vi "jsonToLibera.vi"(0 "json":string, 2 "Enable ADC SP":bool, 5 "Enable DD":bool, 7 "Enable SA":bool, 9 "Enable ADC CW":bool, 13 "Enable AVG":bool) -> (1 "ADC_CW":T1(array[cluster]), 3 "DD":T5(array[cluster]), 4 "mode":i32, 6 "acquisitions":string, 8 "libera_error":i32, 10 "samples":i32, 11 "STATUS":string, 12 "AVG":cluster{"AVG":i32}[](array[cluster]), 14 "SA":T3(array[cluster]), 15 "ADC_SP":T2(array[cluster]))   [LabVIEW 2012]
uses:
  chaos-common-crest/LabVIEW/LV14/chaosui-crest/chaosui-crest.lvlib
panel:
  out "value":T4
  out "nok":i32
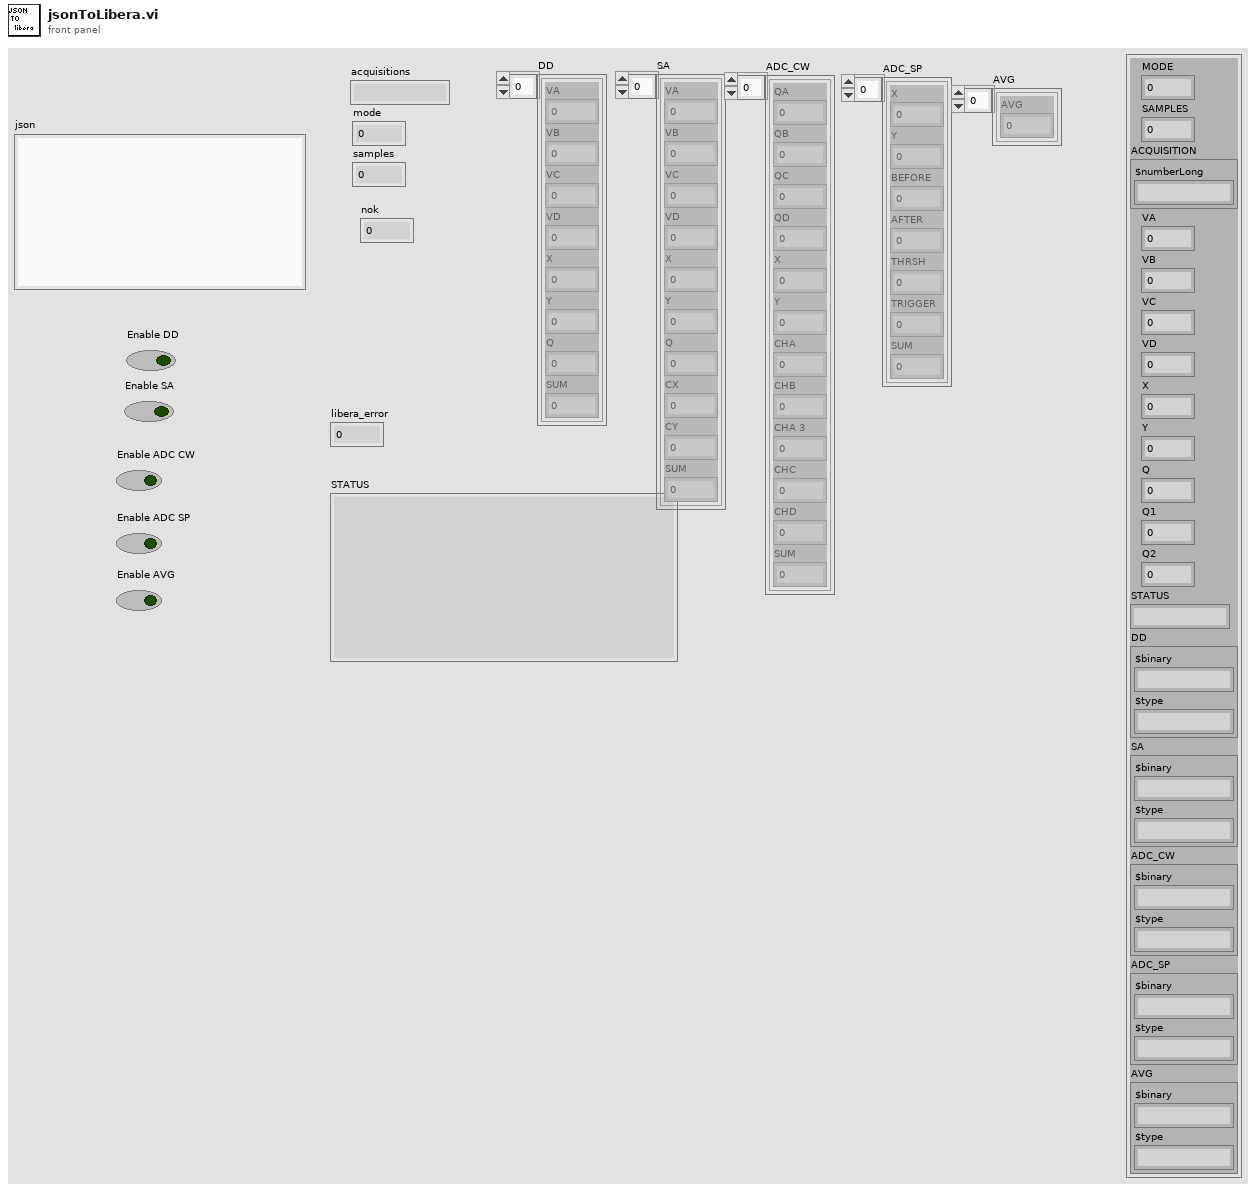
[diagram p1: front panel]
types:
  T1 = cluster{"QA":i32, "QB":i32, "QC":i32, "QD":i32, "X":i32, "Y":i32, "CHA":i32, "CHB":i32, "CHA 3":i32, "CHC":i32, "CHD":i32, "SUM":i32}[]
  T2 = cluster{"X":i32, "Y":i32, "BEFORE":i32, "AFTER":i32, "THRSH":i32, "TRIGGER":i32, "SUM":i32}[]
  T3 = cluster{"VA":i32, "VB":i32, "VC":i32, "VD":i32, "X":i32, "Y ":i32, "Q":i32, "CX":i32, "CY":i32, "SUM":i32}[]
  T4 = cluster{"MODE":i32, "SAMPLES":i32, "ACQUISITION":cluster{"$numberLong":string}, "VA":i32, "VB":i32, "VC":i32, "VD":i32, "X":i32, "Y ":i32, "Q":i32, "Q1":i32, "Q2":i32, "STATUS":string, "DD":cluster{"$binary":string, "$type":string}, "SA":cluster{"$binary":string, "$type":string}, "ADC_CW":cluster{"$binary":string, "$type":string}, "ADC_SP":cluster{"$binary":string, "$type":string}, "AVG":cluster{"$binary":string, "$type":string}}
  T5 = cluster{"VA":i32, "VB":i32, "VC":i32, "VD":i32, "X":i32, "Y ":i32, "Q":i32, "SUM":i32}[]
  T6 = cluster{"MODE":i32, "SAMPLES":i32, "VA":i32, "VB":i32, "VC":i32, "VD":i32, "X":i32, "Y":i32, "ACQUISITION":cluster{"$numberLong":string}, "Q":i32, "STATUS":string, "Q1":i32, "Q2":i32, "DD":cluster{"$binary":string, "$type":string}, "SA":cluster{"$binary":string, "$type":string}, "ADC_CW":cluster{"$binary":string, "$type":string}, "ADC_SP":cluster{"$binary":string, "$type":string}, "AVG":cluster{"$binary":string, "$type":string}, "error":i32}
  T7 = enum16{"big-endian, network order", "native, host order", "little-endian"}
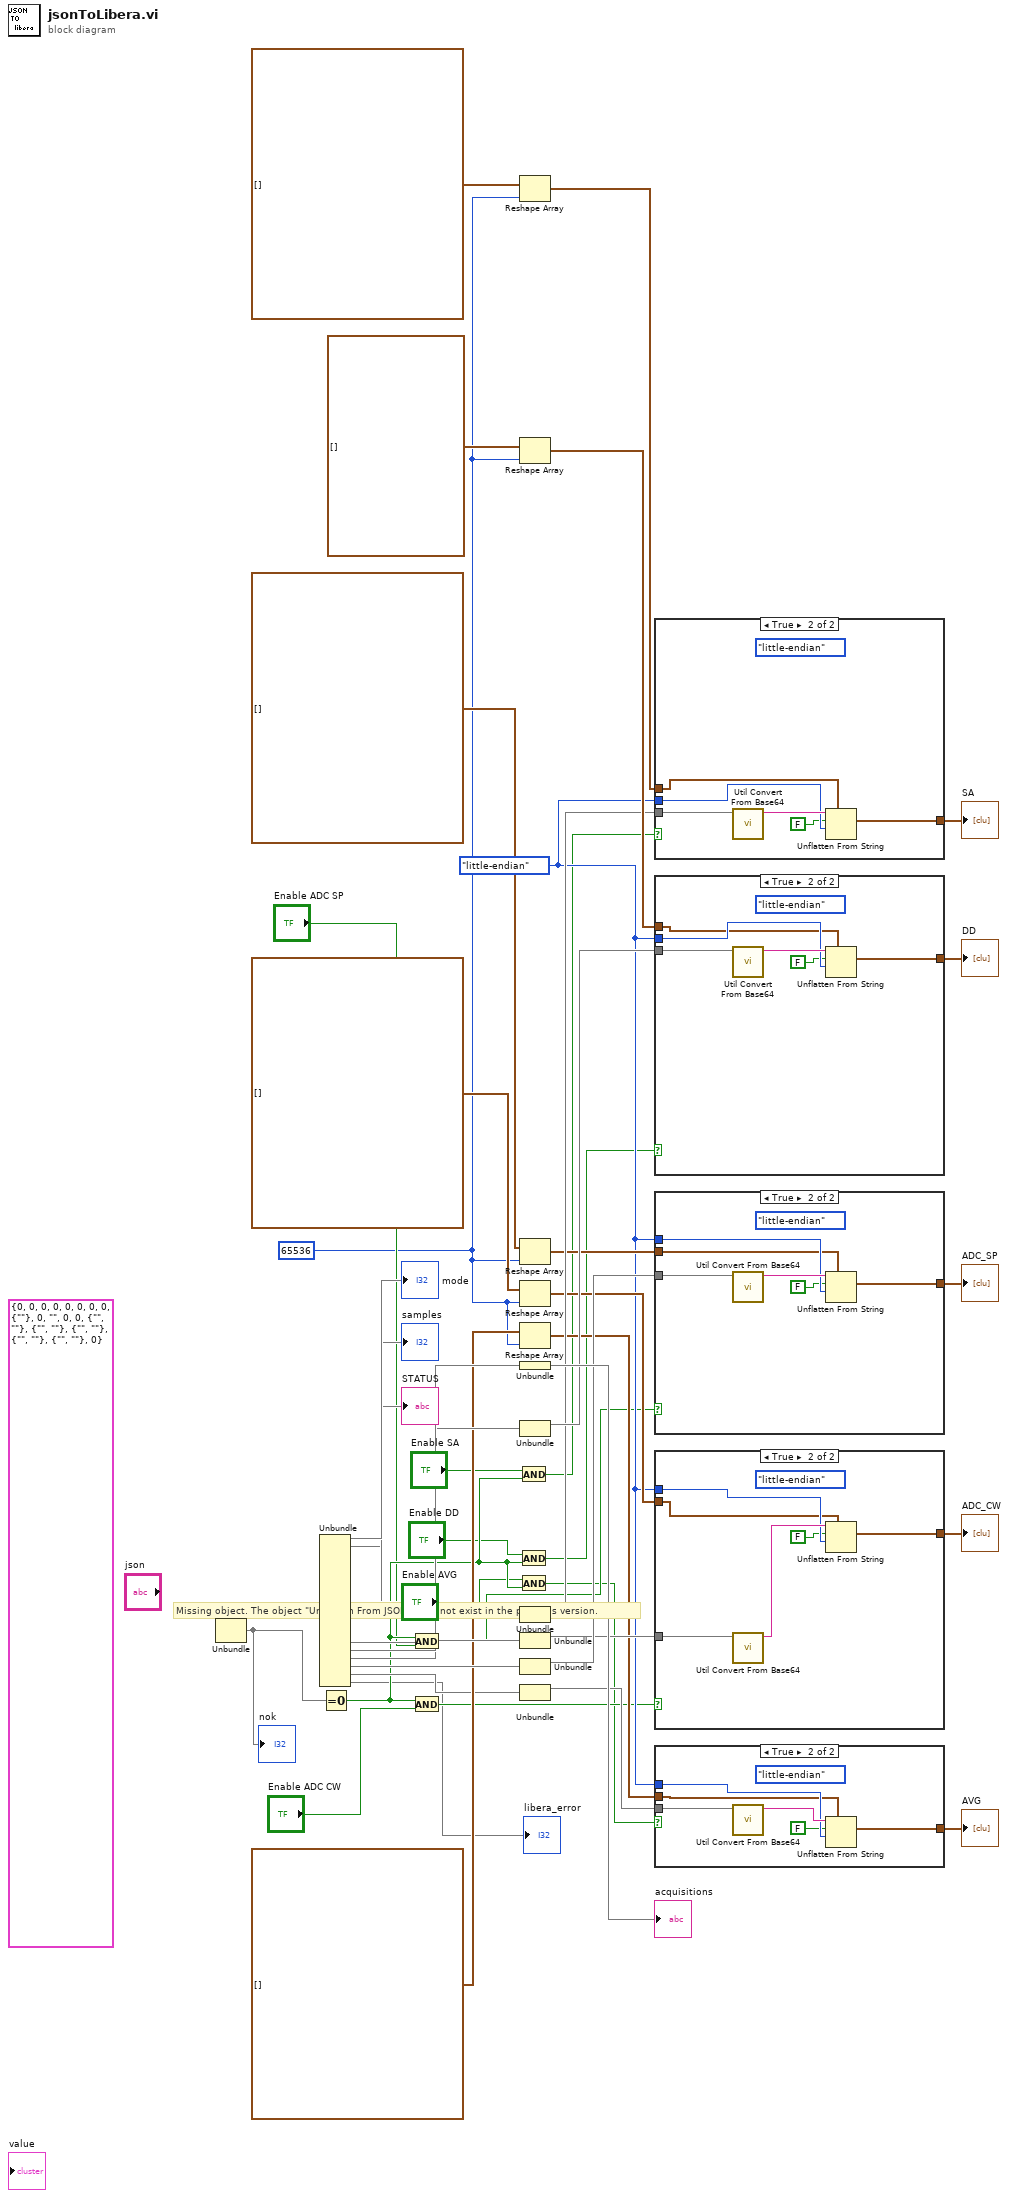
[diagram p0: block diagram]
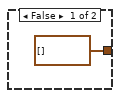
[diagram p2: hidden frame]
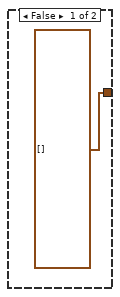
[diagram p3: hidden frame]
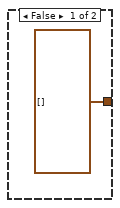
[diagram p4: hidden frame]
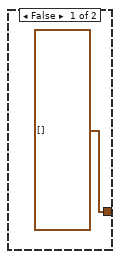
[diagram p5: hidden frame]
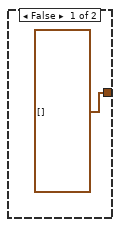
[diagram p6: hidden frame]
diagram:
  w2 = 65536 ("dimension size")
  w43 = T6 {"MODE"=0, "SAMPLES"=0, "VA"=0, "VB"=0, "VC"=0, "VD"=0, "X"=0, "Y"=0, "ACQUISITION"={"$numberLong"=""}, "Q"=0, "STATUS"="", "Q1"=0, "Q2"=0, "DD"={"$binary"="", "$type"=""}, "SA"={"$binary"="", "$type"=""}, "ADC_CW"={"$binary"="", "$type"=""}, "ADC_SP"={"$binary"="", "$type"=""}, "AVG"={"$binary"="", "$type"=""}, "error"=0} ("jsonCluster")
  w18 = T7."little-endian" ("byte order (0:big-endian, network order)")
  # "Missing object. The object \"Unflatten From JSON\" does not exist in the previous version."
  n1 = Unbundle() -> ("code"=w44)  [unwired: 1 in, 2 out]
  "nok" <- w44
  n2 = Unbundle() -> (w47:T6, "MODE"=→"mode", "SAMPLES"=→"samples", "ACQUISITION"=w42, "STATUS"=→"STATUS", "DD"=w40, "SA"=w35, "ADC_CW"=w22, "ADC_SP"=w28, "AVG"=w17, "error"=→"libera_error")  [unwired: 9 out]
  n3 = Equal To 0?(x=w44) -> (x = 0?=w13:bool)
  n4 = And(x=w13, y="Enable ADC SP") -> (x .and. y?=w8:bool)
  n5 = And(x=w13, y="Enable ADC CW") -> (x .and. y?=w6:bool)
  n6 = And(x="Enable SA", y=w13) -> (x .and. y?=w12:bool)
  n7 = And(x="Enable DD", y=w13) -> (x .and. y?=w10:bool)
  n8 = And(x="Enable AVG", y=w13) -> (x .and. y?=w4:bool)
  n9 = Reshape Array(T3 [], w2) -> (w32:T3)
  n10 = Reshape Array(T5 [], w2) -> (w37:T5)
  n11 = Reshape Array(T2 [], w2) -> (w30:T2)
  n12 = Reshape Array(T1 [], w2) -> (w25:T1)
  n13 = Reshape Array(cluster{"AVG":i32}[] [], w2) -> (w20:cluster{"AVG":i32}[])
  n14 = Unbundle(w42) -> (→"acquisitions")
  n15 = Unbundle(w40) -> (w39)  [unwired: 1 out]
  n16 = Unbundle(w35) -> (w34)  [unwired: 1 out]
  n17 = Unbundle(w22) -> (w24)  [unwired: 1 out]
  n18 = Unbundle(w28) -> (w27)  [unwired: 1 out]
  n19 = Unbundle(w17) -> (w16)  [unwired: 1 out]
  n20 = case shown="True" w12 {
    tunnel: w18 -> [_ w53]
    tunnel: w32 -> [_ w52]
    tunnel: [T3 [] w51] -> w31
    tunnel: w34 -> [_ w49]
    frame False {
    }
    frame True {
      (unwired) T7."little-endian" ("byte order (0:big-endian, network order)")
      n21 = call "Util Convert From Base64.vi"("Base64 String"=w49) -> ("String"=w54:string)  [unwired: 9 in, 1 out]
      n22 = Unflatten From String(type=w52, binary string=w54, data includes array or string size? (T)=FALSE, byte order (0:big-endian, network order)=w53) -> (value=w51:T3)  [unwired: 1 in, 2 out]
    }
  }
  "SA" <- w31
  n23 = case shown="True" w10 {
    tunnel: w18 -> [_ w60]
    tunnel: w37 -> [_ w59]
    tunnel: [T5 [] w58] -> w45
    tunnel: w39 -> [_ w57]
    frame False {
    }
    frame True {
      (unwired) T7."little-endian" ("byte order (0:big-endian, network order)")
      n24 = call "Util Convert From Base64.vi"("Base64 String"=w57) -> ("String"=w61:string)  [unwired: 9 in, 1 out]
      n25 = Unflatten From String(type=w59, binary string=w61, data includes array or string size? (T)=FALSE, byte order (0:big-endian, network order)=w60) -> (value=w58:T5)  [unwired: 1 in, 2 out]
    }
  }
  "DD" <- w45
  n26 = case shown="True" w8 {
    tunnel: w18 -> [_ w67]
    tunnel: w30 -> [_ w66]
    tunnel: w27 -> [_ w64]
    tunnel: [T2 [] w63] -> w26
    frame False {
    }
    frame True {
      (unwired) T7."little-endian" ("byte order (0:big-endian, network order)")
      n27 = call "Util Convert From Base64.vi"("Base64 String"=w64) -> ("String"=w68:string)  [unwired: 9 in, 1 out]
      n28 = Unflatten From String(type=w66, binary string=w68, data includes array or string size? (T)=FALSE, byte order (0:big-endian, network order)=w67) -> (value=w63:T2)  [unwired: 1 in, 2 out]
    }
  }
  "ADC_SP" <- w26
  n29 = case shown="True" w6 {
    tunnel: w18 -> [_ w74]
    tunnel: w25 -> [_ w73]
    tunnel: w24 -> [_ w71]
    tunnel: [T1 [] w70] -> w21
    frame False {
    }
    frame True {
      (unwired) T7."little-endian" ("byte order (0:big-endian, network order)")
      n30 = call "Util Convert From Base64.vi"("Base64 String"=w71) -> ("String"=w75:string)  [unwired: 9 in, 1 out]
      n31 = Unflatten From String(type=w73, binary string=w75, data includes array or string size? (T)=FALSE, byte order (0:big-endian, network order)=w74) -> (value=w70:T1)  [unwired: 1 in, 2 out]
    }
  }
  "ADC_CW" <- w21
  n32 = case shown="True" w4 {
    tunnel: w18 -> [_ w81]
    tunnel: w20 -> [_ w80]
    tunnel: w16 -> [_ w78]
    tunnel: [cluster{"AVG":i32}[] [] w77] -> w15
    frame False {
    }
    frame True {
      (unwired) T7."little-endian" ("byte order (0:big-endian, network order)")
      n33 = call "Util Convert From Base64.vi"("Base64 String"=w78) -> ("String"=w82:string)  [unwired: 9 in, 1 out]
      n34 = Unflatten From String(type=w80, binary string=w82, data includes array or string size? (T)=FALSE, byte order (0:big-endian, network order)=w81) -> (value=w77:cluster{"AVG":i32}[])  [unwired: 1 in, 2 out]
    }
  }
  "AVG" <- w15
